vi "Filter.vi"(5 "scope":T2, 7 "error list":variant, 8 "error in (no error)":errorcluster, 10 "filter string":string, 11 "displayed errors in":T1[](array[typedef])) -> (0 "error out":errorcluster, 3 "displayed errors out":T1[](array[typedef]))   [LabVIEW 2017]
uses:
  Error List/Scope.ctl
  Error List/Error Owner and ID.ctl
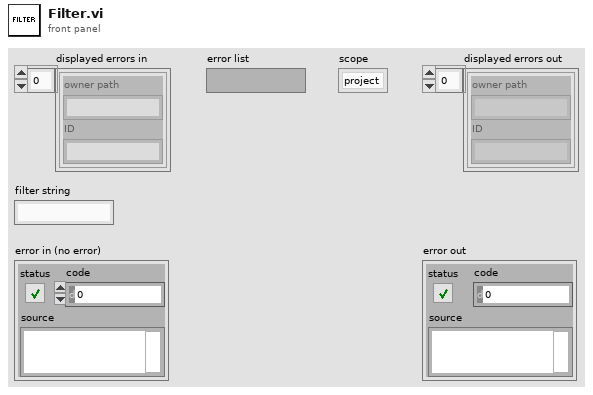
[diagram p1: front panel]
types:
  T1 = typedef "Error Owner and ID.ctl" = cluster{"owner path":string, "ID":string}
  T2 = typedef "Scope.ctl" = enum16{"project", "global"}
  T3 = typedef "Search Query Type.ctl" = enum16{"single code", "code range", "keywords", "error"}
  T4 = typedef "Error File Management.lvlib/NI Error.ctl" = errorcluster
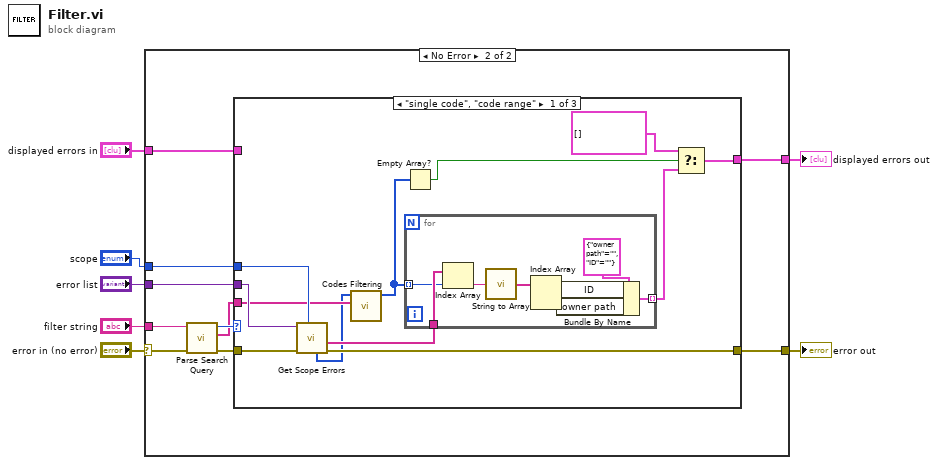
[diagram p0: block diagram]
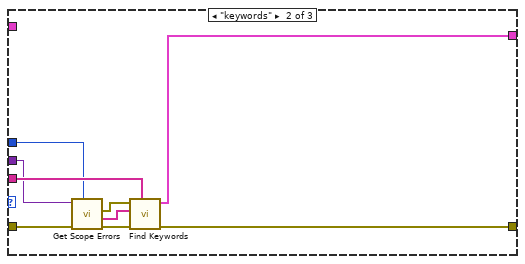
[diagram p3: hidden frame]
diagram:
  n1 = case shown="No Error" "error in (no error)" {
    selector: "error in (no error)" -> [w8 w9]
    tunnel: "scope" -> [_ w18]
    tunnel: "error list" -> [_ w17]
    tunnel: [_ w16] -> w5
    tunnel: "displayed errors in" -> [_ w15]
    tunnel: "filter string" -> [_ w11]
    tunnel: [w8 w10] -> w1
    frame Error {
    }
    frame No Error {
      n2 = call "Parse Search Query.vi"("error in (no error)"=w9, "input string"=w11) -> ("error out"=w12:errorcluster, "searched objects"=w13:string[], "search query"=w14:T3)  [unwired: 7 in]
      n3 = case shown="\"single code\", \"code range\"" w14 {
        tunnel: w13 -> [w21 w47 _]
        tunnel: w12 -> [w27 w46 w49]
        tunnel: [w30 w40 w49] -> w10
        tunnel: [w28 w39 w48] -> w16
        tunnel: w15 -> [_ _ w48]
        tunnel: w17 -> [w26 w44 _]
        tunnel: w18 -> [w25 w43 _]
        frame "single code", "code range" {
          n4 = call "Get Scope Errors.vi"("scope"=w25, "error in (no error)"=w27, "error list <top> in"=w26) -> ("error out"=w30:errorcluster, "attributes"=w24:string[], "error codes"=w20:i32[])  [unwired: 4 in, 2 out]
          n5 = call "Codes Filtering.vi"("searched objects"=w21, "scope error codes"=w20) -> ("found codes indices"=w19:i32[])  [unwired: 9 in]
          n6 = Empty Array?(array=w19) -> (empty?=w29:bool)
          n7 = for {
            tunnel: w24 -> [w38]
            tunnel: w19 -> [w37] mode=indexing
            tunnel: [w33] -> w23 mode=indexing
            n8 = Index Array(array=w38, index=w37) -> (element=w32:string)
            n9 = call "String to Array.vi"("string"=w32) -> ("array"=w36:string[])  [unwired: 1 in]
            n10 = Index Array(array=w36) -> (element #1=w35:string, element #2=w34:string)  [unwired: 2 in]
            n11 = Bundle By Name(cluster=T1 {"owner path"="", "ID"=""} ("owner error"), "ID"=w35, "owner path"=w34) -> (w33:T1)
          }
          n12 = Select(t=T1[] [], s=w29, f=w23) -> (s? t:f=w28:T1[])
        }
        frame "keywords" {
          n13 = call "Get Scope Errors.vi"("scope"=w43, "error in (no error)"=w46, "error list <top> in"=w44) -> ("error out"=w45:errorcluster, "attributes"=w41:string[], "errors"=w42:T4[])  [unwired: 4 in, 2 out]
          n14 = call "Find Keywords.vi"("searched objects"=w47, "error in (no error)"=w45, "attributes"=w41, "errors"=w42) -> ("error out"=w40:errorcluster, "filtered IDs"=w39:T1[])  [unwired: 6 in]
        }
        frame "error" {
        }
      }
    }
  }
  "displayed errors out" <- w5
  "error out" <- w1
